vi "Close serial port.vi"(8 "Error in":errorcluster, 11 "VISA resource name":refnum<visa-resource-name>) -> (0 "Error out":errorcluster)   [LabVIEW 2018]
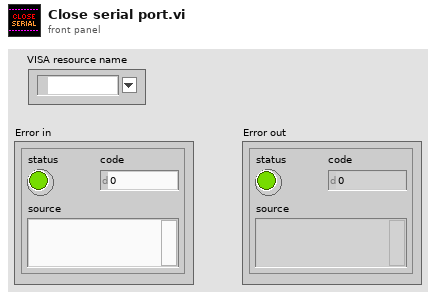
[diagram p1: front panel]
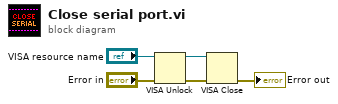
[diagram p0: block diagram]
diagram:
  n1 = VISA Unlock(8:"Error in", 11:"VISA resource name") -> (0:w5:errorcluster, 3:w4:refnum<visa-resource-name>)
  n2 = VISA Close(VISA resource name=w4, error in (no error)=w5) -> (error out=→"Error out":errorcluster)
